vi "MyFPGA Encoder Split Control Lines.vi"(11 "Control":u8 format="%08b") -> (0 "Clear Error?":bool, 1 "Dir/Clock Mode?":bool, 2 "Reset?":bool, 3 "Enable?":bool, 4 "Clear Overflow?":bool)   [LabVIEW 2019]
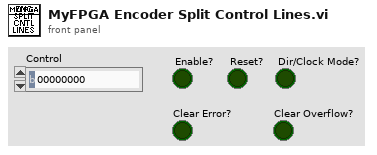
[diagram p1: front panel]
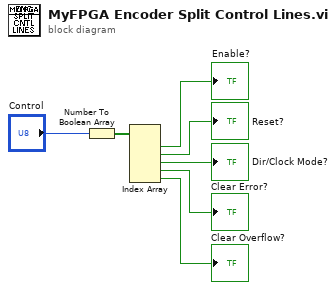
[diagram p0: block diagram]
diagram:
  n1 = Number To Boolean Array(number="Control") -> (Boolean array=w5:bool[])
  n2 = Index Array(array=w5) -> (element #1=→"Enable?":bool, element #2=→"Reset?":bool, element #3=→"Dir/Clock Mode?":bool, element #4=→"Clear Error?":bool, element #5=→"Clear Overflow?":bool)  [unwired: 5 in]
